vi "Down.vi"(2 "背景":dbl[][](array[numeric]), 3 "方块":dbl[][](array[numeric]), 4 "point":cluster{"x":i16, "y":i16} caption="位置") -> (0 "point 2":cluster{"x":i16, "y":i16} caption="新位置", 1 "Landed":bool)   [LabVIEW 2014]
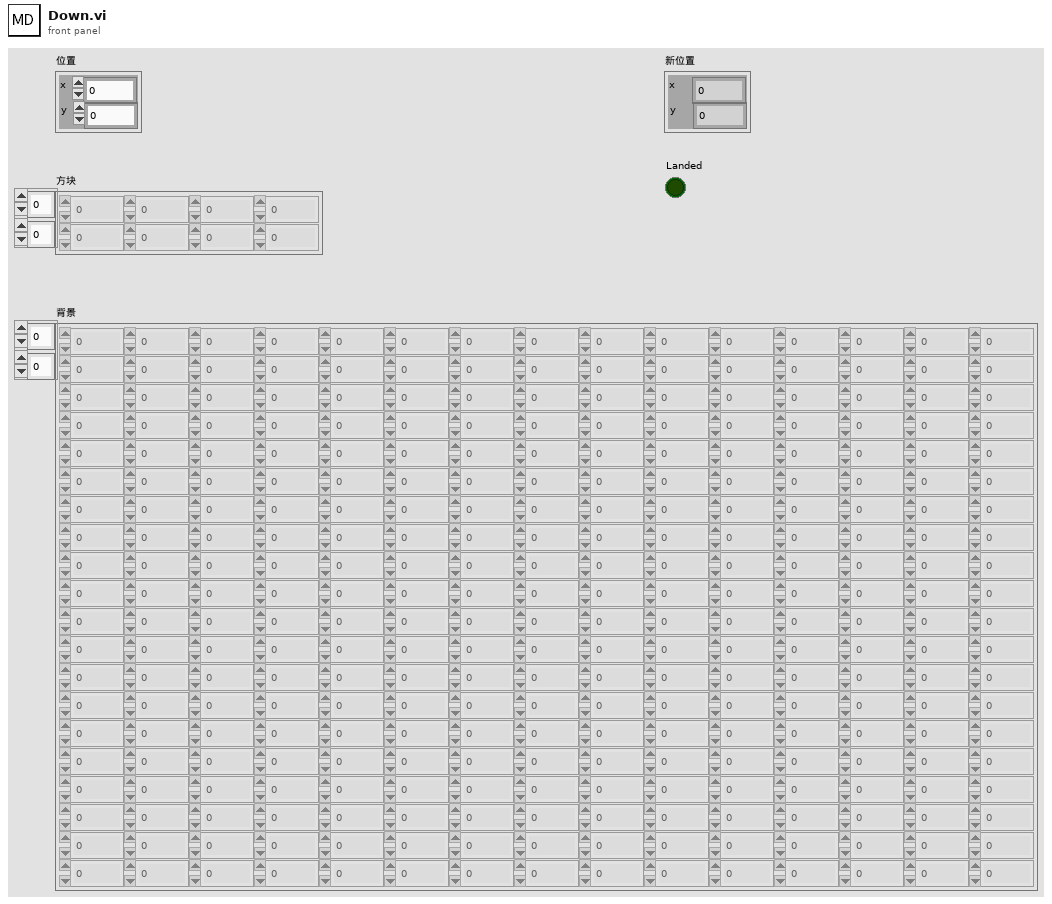
[diagram p1: front panel]
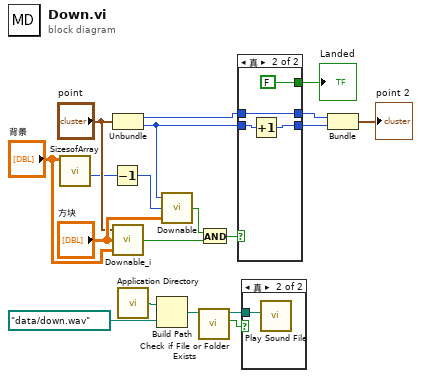
[diagram p0: block diagram]
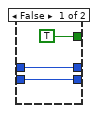
[diagram p3: hidden frame]
diagram:
  n1 = call "SizesofArray.vi"("数组"="背景") -> ("NumRows_r"=w1:i32)  [unwired: 7 in, 3 out]
  n2 = Decrement(x=w1) -> (x-1=w8:i32)
  n3 = Unbundle("point") -> ("x"=w13:i16, "y"=w14:i16)
  n4 = call "Downable_i.vi"("背景"="背景", "方块"="方块", "point"="point") -> ("输出"=w17:bool)
  n5 = call <vilib>:"Application Directory.vi"() -> ("Application Directory"=w6:path)
  n6 = Build Path(base path=w6, name or relative path=path "data/down.wav") -> (appended path=w5:path)
  n7 = call "Downable.vi"("输入"="方块", "Bottom"=w8, "y"=w14) -> ("输出"=w18:bool)
  n8 = call <vilib>:"Check if File or Folder Exists.vi"("path"=w5) -> ("file or folder exists?"=w4:bool, "dup path"=w3:path)  [unwired: 8 in, 1 out]
  n9 = And(x=w18, y=w17) -> (x .and. y?=w16:bool)
  n10 = case shown="真" w16 {
    tunnel: w14 -> [w21 w26]
    tunnel: w13 -> [w22 w25]
    tunnel: [w22 w25] -> w12
    tunnel: [w21 w24] -> w11
    tunnel: [TRUE FALSE] -> w9
    frame False {
    }
    frame True {
      n11 = Increment(x=w26) -> (x+1=w24:i16)
    }
  }
  "Landed" <- w9
  n12 = case shown="真" w4 {
    tunnel: w3 -> [_ w27]
    frame False {
    }
    frame True {
      n13 = call <vilib>:"Play Sound File.vi"("path"=w27) -> ()  [unwired: 9 in, 2 out]
    }
  }
  n14 = Bundle("x"=w12, "y"=w11) -> (→"point 2":cluster{"x":i16, "y":i16})  [unwired: 1 in]
